vi "test Get and Set Transfer Groups.vi"(8 "error in (no error)":errorcluster, 11 "TestCase in":refnum<class "Framework Tests.lvclass">) -> (0 "error out":errorcluster, 3 "TestCase out":refnum<class "Framework Tests.lvclass">)   [LabVIEW 2017, in "Framework Tests.lvclass"]
uses:
  Framework Tests.lvclass
  Engine/Classes/Transfer Group/Transfer Group.lvclass
  Mock Framework Class/Mock Framework.lvclass
  C:/github/data-sharing-framework/Data Sharing Framework Core/Engine/Classes/Framework/Framework.lvclass
  Engine/Classes/Framework/Framework.lvclass/Framework.ctl
  <vilib>/addons/_JKI Toolkits/VI Tester/TestCase.llb/TestCase.lvclass
  Engine/Classes/Framework/Framework.lvclass
  C:/Program Files (x86)/National Instruments/LabVIEW 2017/vi.lib/addons/_JKI Toolkits/VI Tester/TestCase.llb/TestCase.lvclass
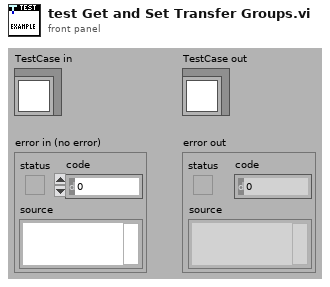
[diagram p1: front panel]
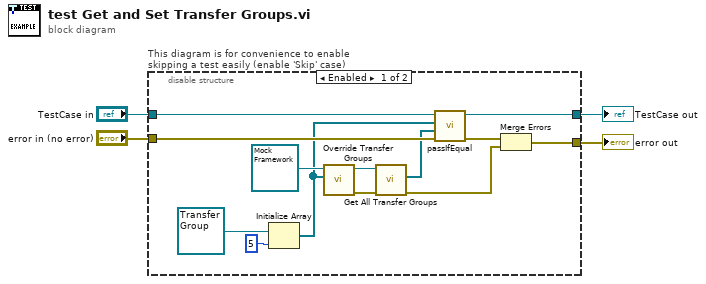
[diagram p0: block diagram]
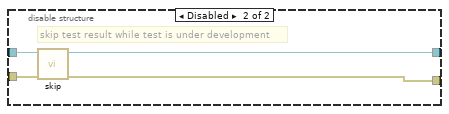
[diagram p2: hidden frame]
diagram:
  n1 = disable-structure "This diagram is for convenience to enable skipping a test easily (enable 'Skip' case)" shown="Enabled" {
    disable-tunnel: "TestCase in" -> [w10 w20]
    disable-tunnel: [w9 w18] -> w1
    disable-tunnel: [w8 w19] -> w3
    disable-tunnel: "error in (no error)" -> [w16 w17]
    frame Enabled {
      n2 = Initialize Array(refnum<class "Transfer Group.lvclass"> refnum ("DSF Core.lvlib:Transfer Group"), 5 ("dimension size")) -> (w6:refnum<class "Transfer Group.lvclass">[])
      n3 = call "Override Transfer Groups.vi"("All Transfers"=w6, "Mock Framework in"=refnum<class "Mock Framework.lvclass"> refnum) -> ("error out"=w7:errorcluster, "Mock Framework out"=w12:refnum<class "Mock Framework.lvclass">)  [unwired: 8 in]
      n4 = call "Get All Transfer Groups.vi"("Framework in"=w12) -> ("All Transfer Groups"=w5:refnum<class "Transfer Group.lvclass">[])  [unwired: 9 in, 1 out]
      n5 = call-dynamic "passIfEqual.vi"("error in (no error)"=w16, "y"=w5, "x"=w6, "TestCase in"=w10) -> ("error out"=w11:errorcluster, "TestCase out"=w9:refnum<class "Framework Tests.lvclass">)  [unwired: 6 in]
      n6 = Merge Errors(w11, w7) -> (w8:errorcluster)
    }
    frame Disabled {
      # "skip test result while test is under development"
      n7 = call <vilib>:"skip.vi"("error in (no error)"=w17, "TestCase in"=w20) -> ("error out"=w19:errorcluster, "TestCase out"=w18:refnum<class "Framework Tests.lvclass">)  [unwired: 8 in]
    }
  }
  "error out" <- w3
  "TestCase out" <- w1
